vi "Update Host Sample Data.vi"(6 "Scan Data Array":u32[](array[numeric]), 7 "InspectCycle":bool, 8 "error in (no error)":errorcluster, 9 "Cancelled":bool, 10 "Success":bool, 11 "Acquiring Data":bool) -> (0 "error out":errorcluster)   [LabVIEW 2015, in "Tool Module.lvlib"]
uses:
  Tool Module.lvlib
  _Sample Data Rtn Cluster--typedef.ctl
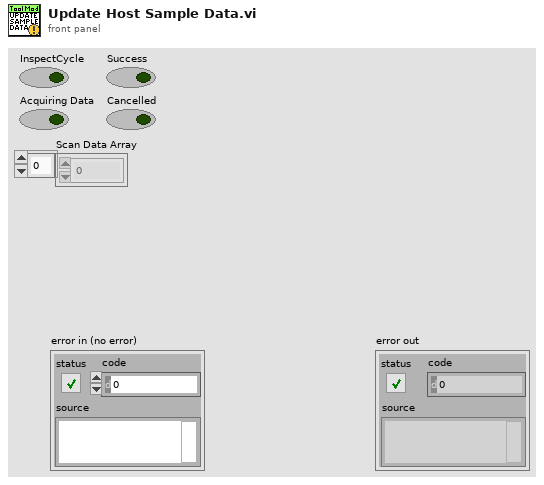
[diagram p1: front panel]
types:
  T1 = typedef "Tool Module.lvlib/_Sample Data Rtn Cluster--typedef.ctl" = cluster{"InspectCycle":bool, "Acquiring Data":bool, "Success":bool, "Cancelled":bool, "Scan Data Array":u32[], "error cluster":errorcluster}
  T2 = typedef "Tool Module.lvlib/_Sample Data Notifier--typedef.ctl" = refnum<notifier>
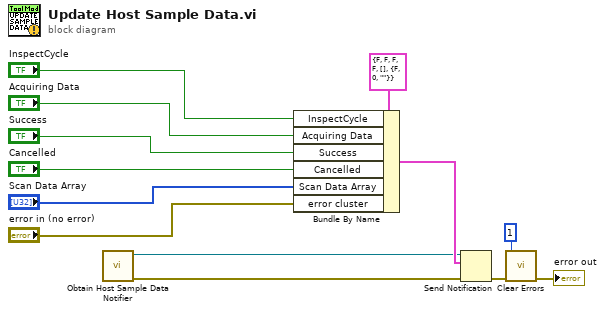
[diagram p0: block diagram]
diagram:
  n1 = call "Obtain Host Sample Data Notifier.vi"() -> ("error out"=w11:errorcluster, "Sample Data Notifier"=w1:T2)  [unwired: 10 in]
  n2 = Bundle By Name(cluster=T1 {"InspectCycle"=FALSE, "Acquiring Data"=FALSE, "Success"=FALSE, "Cancelled"=FALSE, "Scan Data Array"=[], "error cluster"={"status"=FALSE, "code"=0, "source"=""}} ("_Full Scan Data Rtn Cluster"), "InspectCycle"="InspectCycle", "Acquiring Data"="Acquiring Data", "Success"="Success", "Cancelled"="Cancelled", "Scan Data Array"="Scan Data Array", "error cluster"="error in (no error)") -> (w12:T1)
  n3 = Send Notification(notification=w12, notifier=w1, error in (no error)=w11) -> (error out=w5:errorcluster)  [unwired: 1 out]
  n4 = call <vilib>:"Clear Errors.vi"("error in (no error)"=w5, "specific error code to clear (0: all)"=1) -> ("error out"=→"error out":errorcluster)  [unwired: 4 in, 1 out]
